vi "lowLevelControllerPostRun.vi"(8 "error in (no error)":errorcluster) -> (0 "error out":errorcluster)   [LabVIEW 2017, in "lowLevelController.lvlib"]
doc: "This VI releases the Low Level Control Queue."
uses:
  lowLevelController.lvlib
  Queue/TypeDefs/queueFGVState.ctl
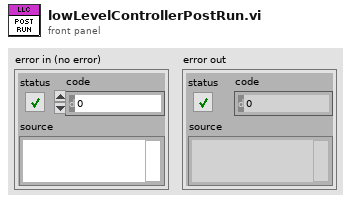
[diagram p1: front panel]
types:
  T1 = typedef "lowLevelController.lvlib/queueFGVState.ctl" = enum16{"set", "get"}
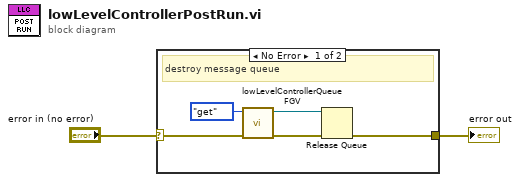
[diagram p0: block diagram]
diagram:
  n1 = case shown="No Error" "error in (no error)" {
    selector: "error in (no error)" -> [w7 w8]
    tunnel: [w4 w8] -> w1
    frame No Error {
      # "destroy message queue"
      n2 = call "lowLevelControllerQueueFGV.vi"("error in (no error)"=w7, 11:queueFGVState."get") -> ("error out"=w5:errorcluster, "queue out"=w3:refnum<queue>)  [unwired: 8 in]
      n3 = Release Queue(queue=w3, error in (no error)=w5) -> (error out=w4:errorcluster)  [unwired: 1 in, 2 out]
    }
    frame Error {
    }
  }
  "error out" <- w1
